vi "Untitled 7 (SubVI).vi"(5 "Dev löschen":bool, 6 "dev id":i32, 7 "reference":refnum<vi>, 8 "error in (no error)":errorcluster, 9 "Elternobjekt-Tag":string, 10 "Tree pics & devs":refnum<vi>, 11 "Device in":refnum<class "Device.lvclass">) -> (0 "error out":errorcluster)   [LabVIEW 2013]
uses:
  classes/Datastructure/Device/Device.lvclass
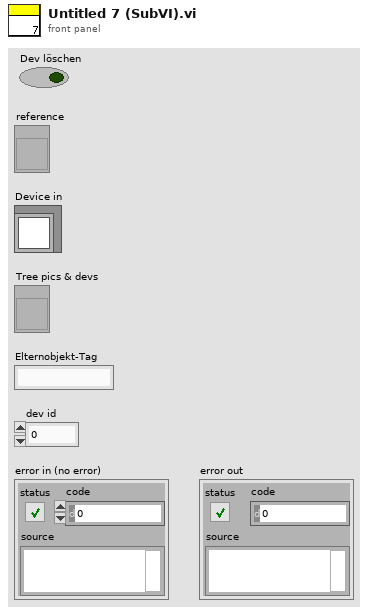
[diagram p1: front panel]
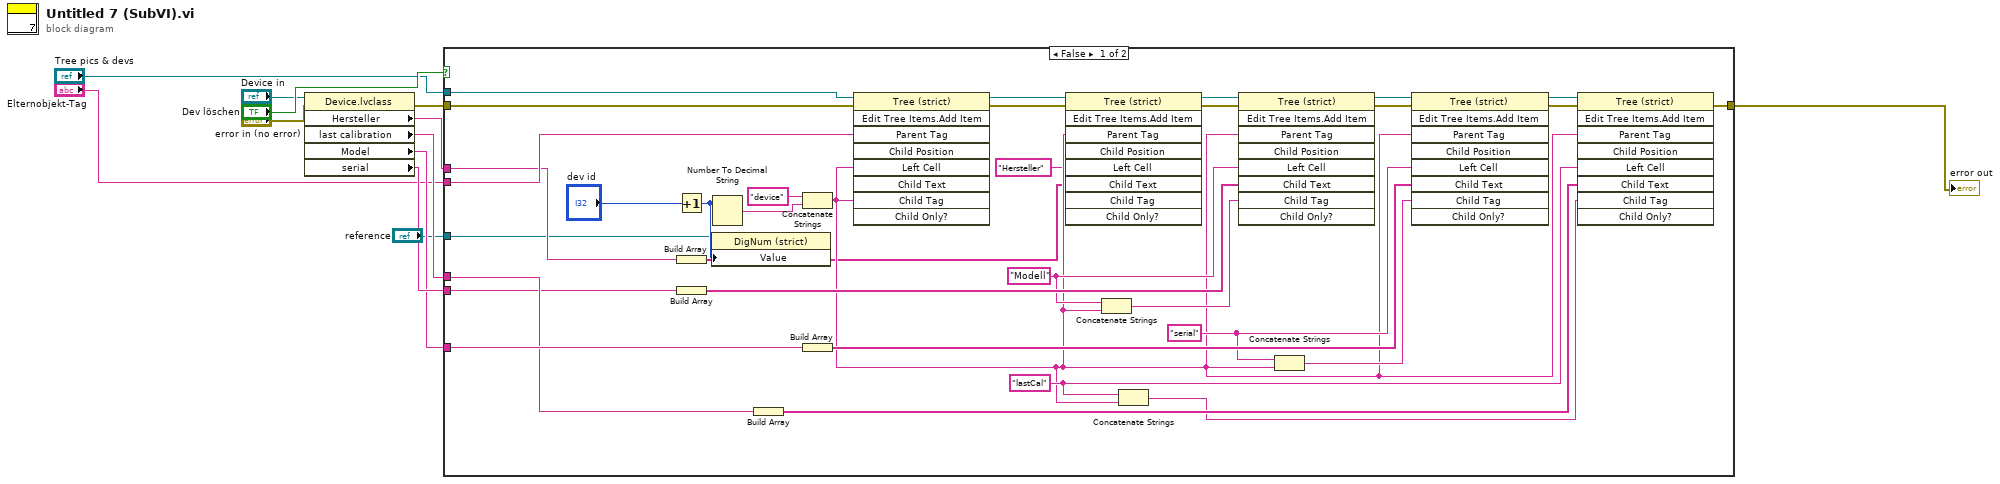
[diagram p0: block diagram]
diagram:
  n1 = property class="Device.lvclass"(reference="Device in", error in="error in (no error)") -> (error out=w9:errorcluster, "Hersteller"=w5:string, "last calibration"=w6:string, "Model"=w7:string, "serial"=w8:string)  [unwired: 1 out]
  n2 = case shown="False" "Dev löschen" {
    tunnel: "Elternobjekt-Tag" -> [w41 _]
    tunnel: w8 -> [w16 _]
    tunnel: w7 -> [w36 _]
    tunnel: w6 -> [w35 _]
    tunnel: [w25 w46] -> w4
    tunnel: "Tree pics & devs" -> [w24 _]
    tunnel: w5 -> [w15 _]
    tunnel: w9 -> [w14 w46]
    tunnel: "reference" -> [w13 _]
    frame False {
      w27 = "lastCal" ("Linker Zellen-String")
      w29 = "serial" ("Linker Zellen-String")
      w31 = "Modell" ("Linker Zellen-String")
      n3 = Increment(x="dev id") -> (x+1=w42:i32)
      n4 = Build Array(w15) -> (w17:string[])
      n5 = Build Array(w16) -> (w34:string[])
      n6 = property class="DigNum (strict)"(reference=w13, "Value"=w42) -> ()  [unwired: 1 in, 2 out]
      n7 = Number To Decimal String(number=w42) -> (decimal integer string=w44:string)  [unwired: 1 in]
      n8 = Build Array(w35) -> (w32:string[])
      n9 = Concatenate Strings("device" ("Left Cell String"), w44) -> (w19:string)
      n10 = Build Array(w36) -> (w33:string[])
      n11 = invoke class="Tree (strict)" method="Edit Tree Items.Add Item"(reference=w24, error in=w14, "Parent Tag"=w41, "Left Cell"=w19, "Child Tag"=w19) -> (reference out=w21:refnum<vi>, error out=w20:errorcluster)  [unwired: 4 in, 7 out]
      n12 = invoke class="Tree (strict)" method="Edit Tree Items.Add Item"(reference=w21, error in=w20, "Parent Tag"=w19, "Left Cell"="Hersteller" ("Left Cell String"), "Child Text"=w17) -> (reference out=w23:refnum<vi>, error out=w22:errorcluster)  [unwired: 4 in, 7 out]
      n13 = Concatenate Strings(w31, w19) -> (w30:string)
      n14 = Concatenate Strings(w27, w19) -> (w26:string)
      n15 = invoke class="Tree (strict)" method="Edit Tree Items.Add Item"(reference=w23, error in=w22, "Parent Tag"=w19, "Left Cell"=w31, "Child Text"=w34, "Child Tag"=w30) -> (reference out=w40:refnum<vi>, error out=w39:errorcluster)  [unwired: 3 in, 7 out]
      n16 = Concatenate Strings(w29, w19) -> (w28:string)
      n17 = invoke class="Tree (strict)" method="Edit Tree Items.Add Item"(reference=w40, error in=w39, "Parent Tag"=w19, "Left Cell"=w29, "Child Text"=w33, "Child Tag"=w28) -> (reference out=w37:refnum<vi>, error out=w38:errorcluster)  [unwired: 3 in, 7 out]
      n18 = invoke class="Tree (strict)" method="Edit Tree Items.Add Item"(reference=w37, error in=w38, "Parent Tag"=w19, "Left Cell"=w27, "Child Text"=w32, "Child Tag"=w26) -> (error out=w25:errorcluster)  [unwired: 3 in, 8 out]
    }
    frame True {
    }
  }
  "error out" <- w4
